vi "Instrument Identification.vi"() -> ()   [LabVIEW 2023]
doc: "Provides an example implementation of the Hardware Abstraction Framework to allow any attached instrument to be queried for its identity. The instrument must implement the SCPI standard.\n\nThe example application is clearly overly complex for the simple purpose of obtaining identity. However, it has been written to show how complex applications can be derived using the provided Event-Process-Result Handling mechanism. In fact, the base application can be reused by replacing the \"App ActionX Process\" VIs and \"Result Handling VIs\" as needed.\n\nNote that this example is just one way of interacting with the Framework. Ultimately, you just need to set up a Test Processor with what is needed and tell it to \"Process Directors\"."
uses:
  ReadCommand/ReadCommand.lvclass
  All Internal Message Ids.ctl
  ResourceEnumerator/ResourceEnumerator.lvclass
  CommandDirector/CommandDirector.lvclass
  TestProcessor/TestProcessor.lvclass
  <extravilib>/ChannelInstances/Tag-bool/Read With Abort.vi
  <extravilib>/ChannelInstances/Tag-bool/Write With Abort.vi
  <extravilib>/ChannelInstances/Tag-bool/Instantiate.vi
  <extravilib>/ChannelInstances/Tag-bool/EndpointRead.vi
  <extravilib>/ChannelInstances/Tag-bool/Endpoint.vi
  HAF.lvlib
  <extravilib>/ChannelInstances/Tag-bool.lvlib
panel:
  out "error out":errorcluster
  out "IDs":string[](array[string])
  out "Running":bool
  in  "Action10":bool
  in  "Action9":bool
  in  "Action8":bool
  in  "Action7":bool
  in  "Action6":bool
  in  "Action5":bool
  in  "Action4":bool
  in  "Action3":bool
  in  "Action2":bool
  in  "Instruments 2":string(combo)
  in  "Resume":bool
  in  "Pause":bool
  in  "Stop":bool
  in  "Get Id":bool caption="Action1"
  out "Instrument Id":string
  in  "Refresh":bool
  in  "Instruments":string(combo)
  # "Defined Behaviour Buttons"
  # "Instrument Identification"
  # "Re-usable Controls\n\nThese are hidden at runtime.  Unhide if used."
  # "Provides an example implementation of the Hardware Abstraction Framework to allow any attached instrument to be queried for its identity.  The instrument must implement the SCPI standard and must be defined in line with those in Implementation>Instrument.\n\nChoose an Instrument from the drop down list and click on Get Id.  The list can be refreshed by clicking Refresh.  The VI is terminated by clicking on Stop.\n\nThe example application is clearly overly complex for the simple purpose of obtaining identity.  However, it has been written to show how complex applications can be derived using the provided Event-Process-Result Handling mechanism.  In fact, the base application can be reused by replacing the \"App ActionX Process\" VIs and \"Result Handling VIs\" as needed.\n\nNote that this example is just one way of interacting with the Framework.  Ultimately, you just need to set up a Test Processor with what is needed and tell it to \"Process Directors\"."
  # "Defined Behaviour Buttons\n\nDrag the control from here to where needed.  You can relabel them but their behaviour is fixed in the application.\nYou may change this behaviour as well of course.\nStop and Refresh have been used."
  # "Instruments"
  # "Action Buttons"
  # "Instruments\n\nThese hold a list of Instruments attached to the PC and are populated by the \"Refresh\" Process case.  The Refresh button re-populates them."
  # "Action  Buttons\n\nDrag the control from here to where you need them on your panel.  Re-label and add button text as desired.\n\nPut processing code in the Process Case under their caption value.\n\nAction1 has been used and named \"Get Id\""
  # "Other"
  # "Other\n\nOther potentially useful controls or indicators. \nIDs is the collection of UUIDs generated for Commands during execution.\nThe LED Running is used in this example."
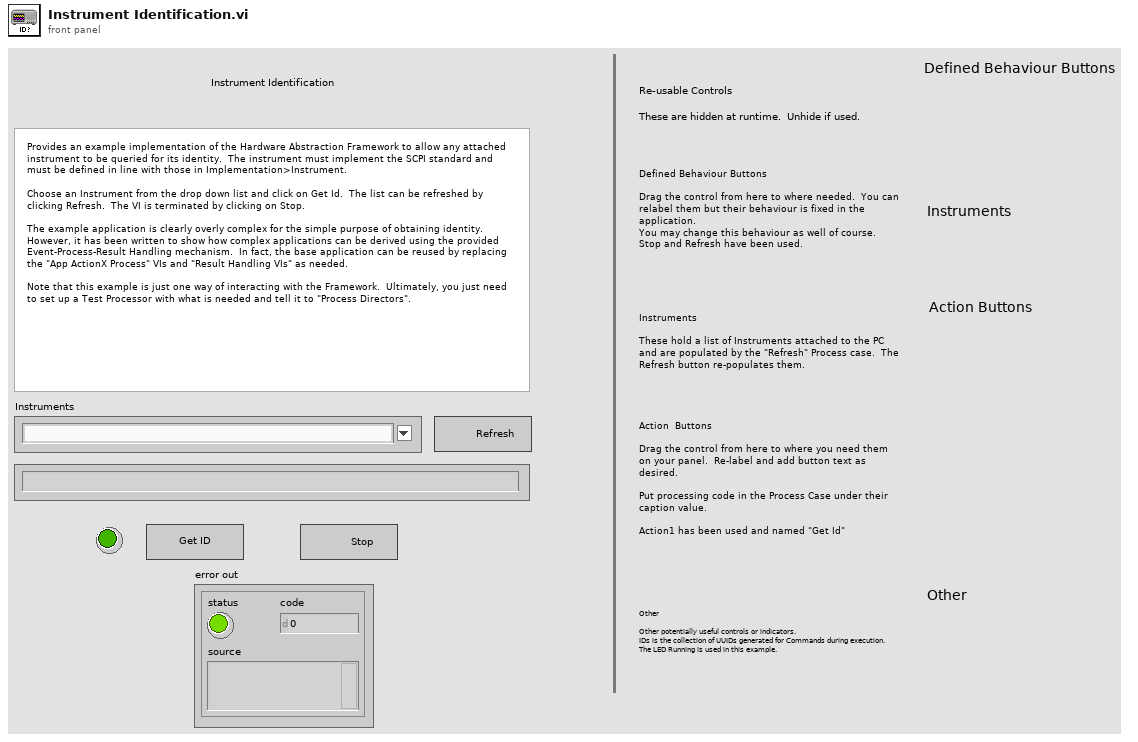
[diagram p1: front panel]
types:
  T1 = typedef "HAF.lvlib/All Message Queues.ctl" = cluster{"Internal":refnum<queue>, "Notifications":refnum<queue>}
  T2 = typedef "HAF.lvlib/All Events.ctl" = cluster{"Stop":T3, "Pause":T4, "Resume":T5, "Done":T6, "Injection":T7}
  T3 = typedef "HAF.lvlib/Stop Event.ctl" = refnum<user-event>
  T4 = typedef "HAF.lvlib/Pause Event.ctl" = refnum<user-event>
  T5 = typedef "HAF.lvlib/Resume Event.ctl" = refnum<user-event>
  T6 = typedef "HAF.lvlib/Done Event.ctl" = refnum<user-event>
  T7 = typedef "HAF.lvlib/Injection Event.ctl" = refnum<user-event>
  T8 = typedef "HAF.lvlib/All Internal Message Ids.ctl" = cluster{"Initialise":string, "Process":string, "Continue":string, "Done":string, "Pause":string, "Resume":string, "Stop":string, "Exit":string, "Inject":string}
  T9 = typedef "Tag-bool.lvlib/))Channel.ctl" = refnum<queue>
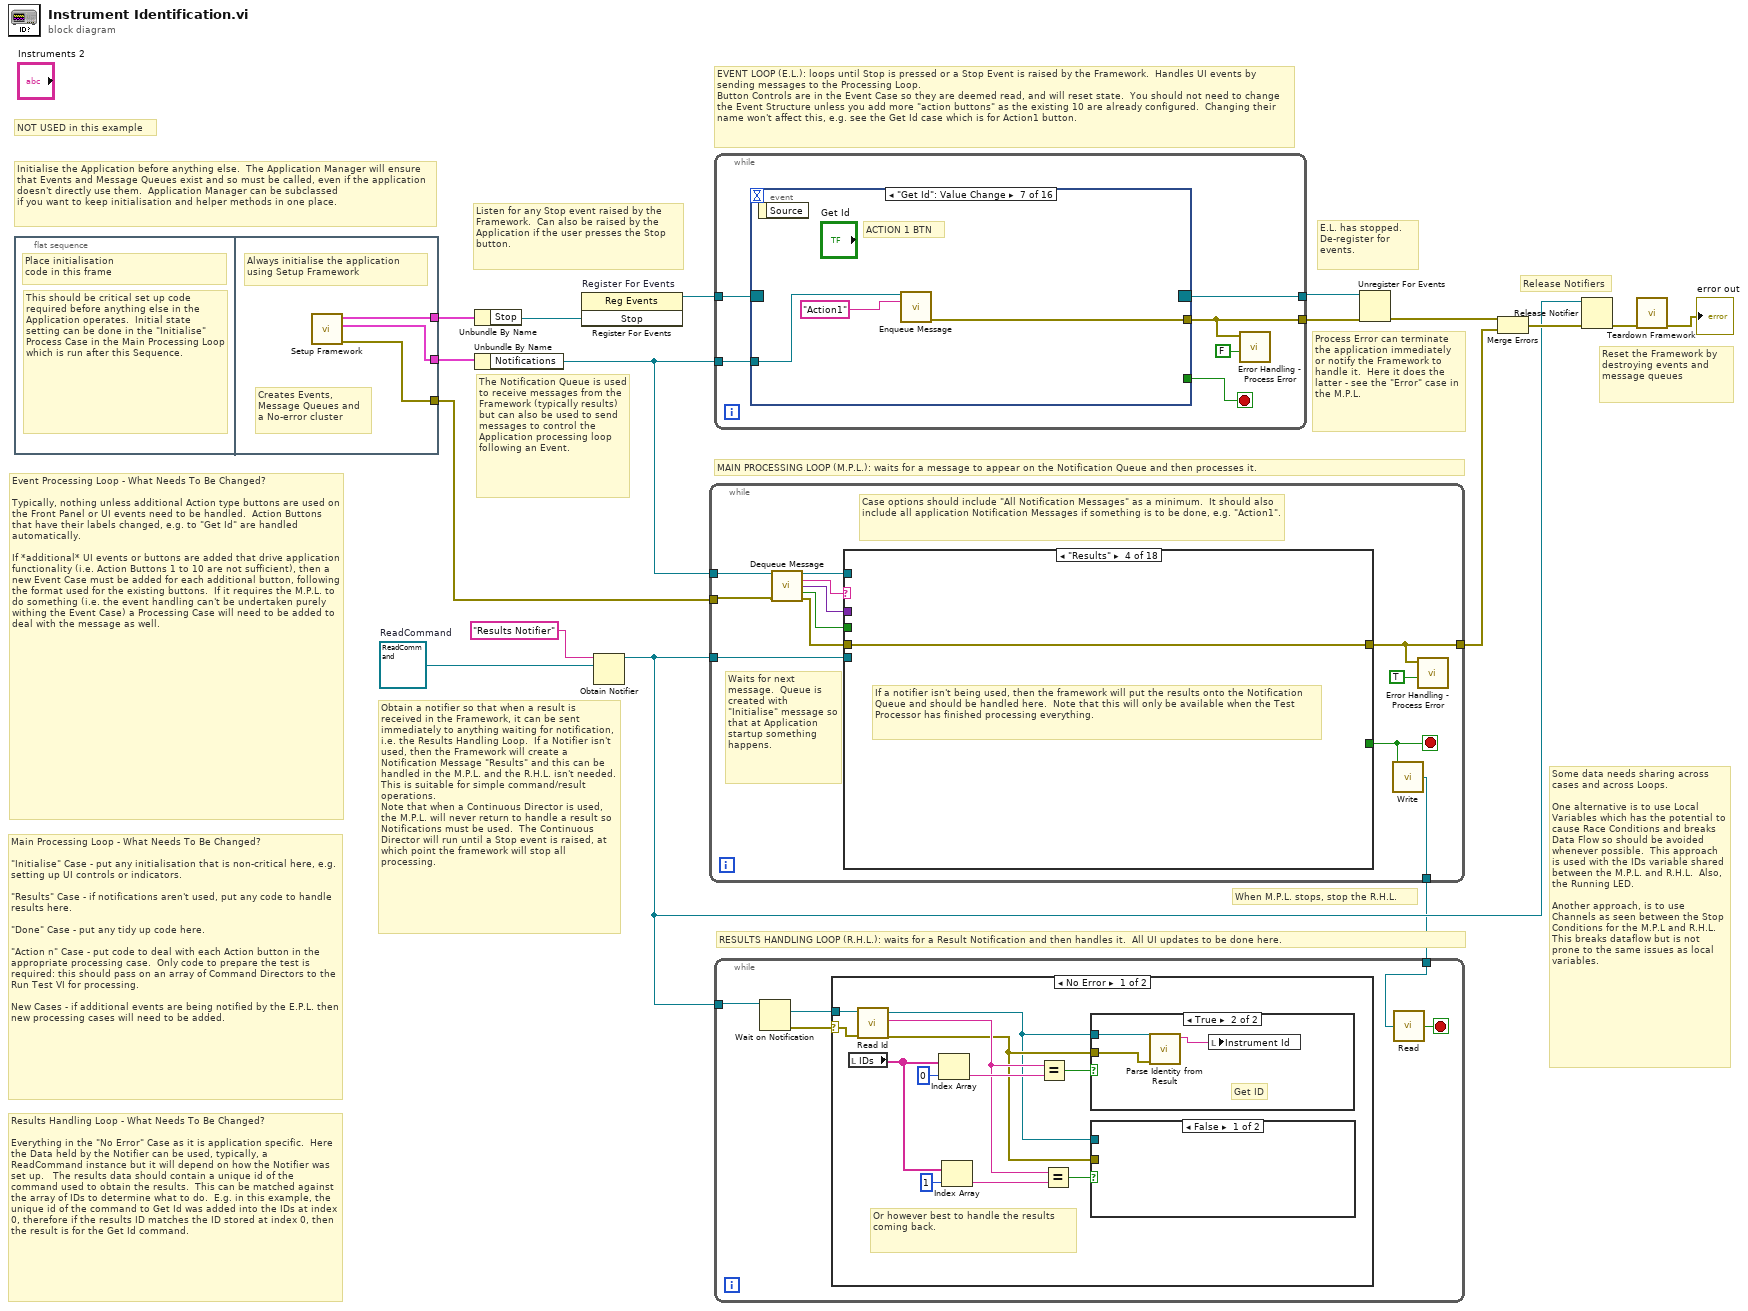
[diagram p0: block diagram]
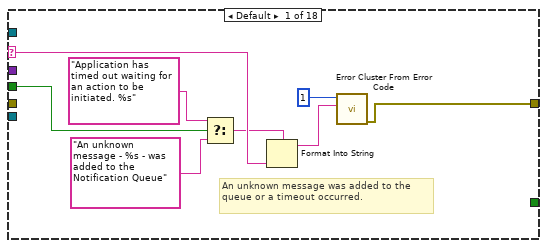
[diagram p5: hidden frame]
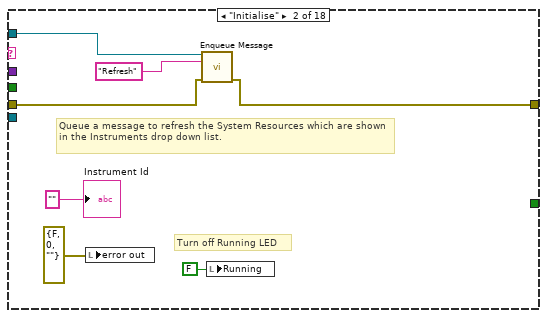
[diagram p6: hidden frame]
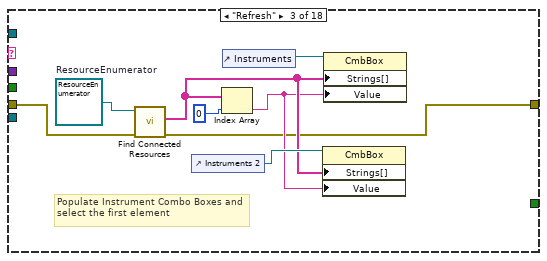
[diagram p7: hidden frame]
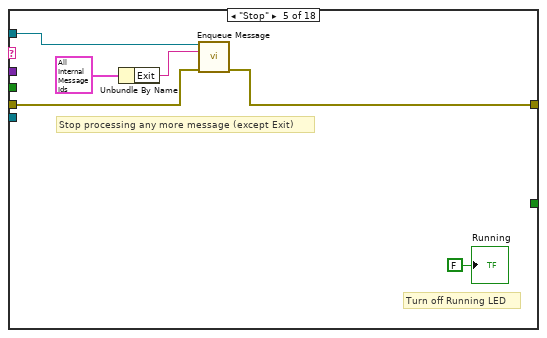
[diagram p8: hidden frame]
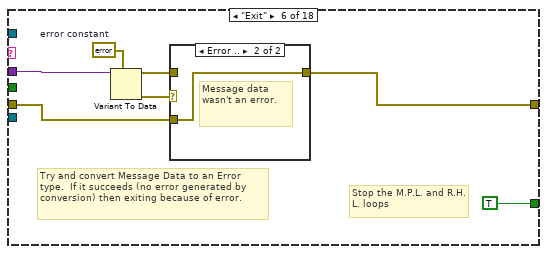
[diagram p9: hidden frame]
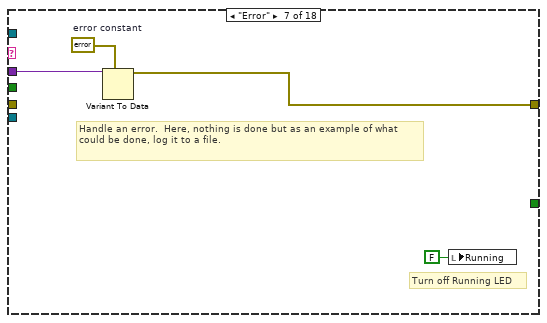
[diagram p11: hidden frame]
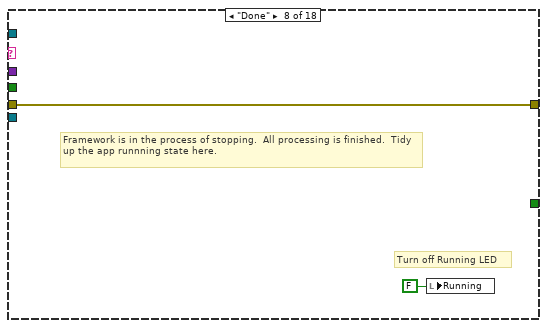
[diagram p12: hidden frame]
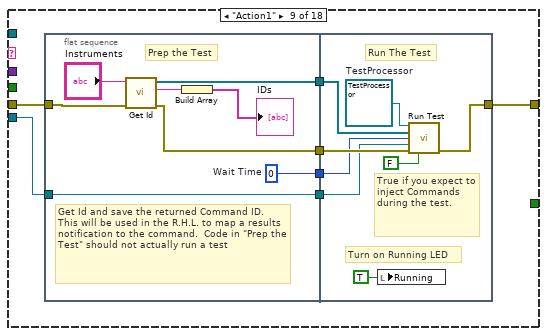
[diagram p13: hidden frame]
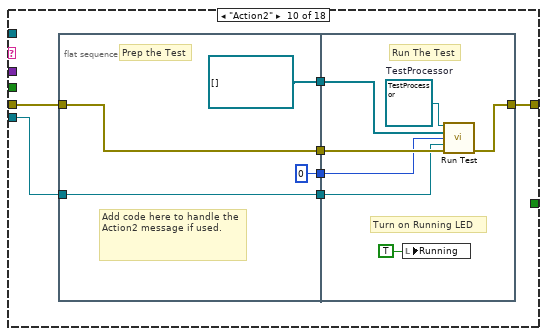
[diagram p14: hidden frame]
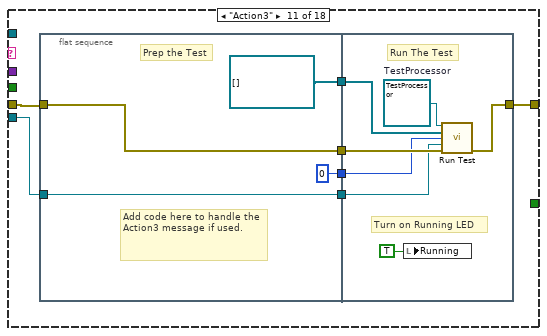
[diagram p15: hidden frame]
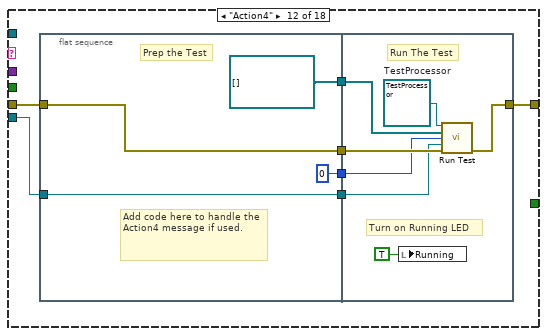
[diagram p16: hidden frame]
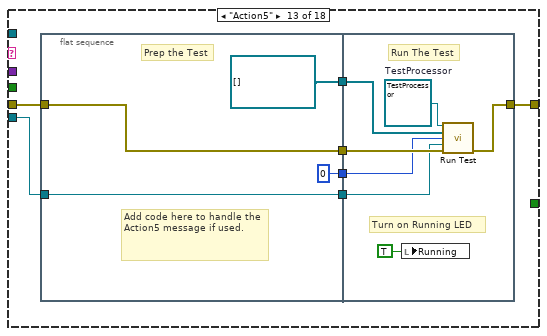
[diagram p17: hidden frame]
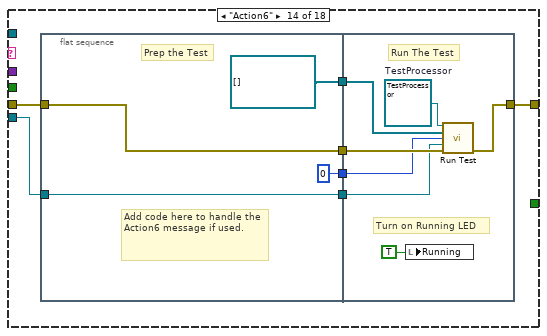
[diagram p18: hidden frame]
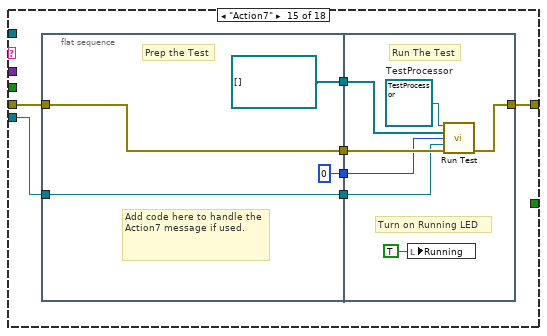
[diagram p19: hidden frame]
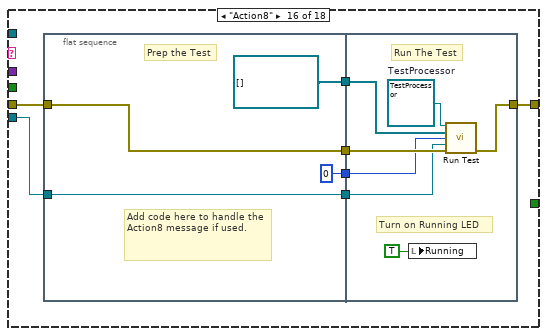
[diagram p20: hidden frame]
diagram:
  w8 = refnum<class "ReadCommand.lvclass"> refnum  # ReadCommand
  # "When M.P.L. stops, stop the R.H.L."
  # "Results Handling Loop - What Needs To Be Changed?\n\nEverything in the \"No Error\" Case as it is application specific.  Here the Data held by the Notifier can be used, typically, a ReadCommand instance but it will depend on how the Notifier was set up.   The results data should contain a unique id of the command used to obtain the results.  This can be matched against the array of IDs to determine what to do.  E.g. in this example, the unique id of the command to Get Id was added into the IDs at index 0, therefore if the results ID matches the ID stored at index 0, then the result is for the Get Id command."
  # "Reset the Framework by destroying events and message queues"
  # "Release Notifiers"
  # "Main Processing Loop - What Needs To Be Changed?\n\n\"Initialise\" Case - put any initialisation that is non-critical here, e.g. setting up UI controls or indicators.\n\n\"Results\" Case - if notifications aren't used, put any code to handle results here.\n\n\"Done\" Case - put any tidy up code here.\n\n\"Action n\" Case - put code to deal with each Action button in the appropriate processing case.  Only code to prepare the test is required: this should pass on an array of Command Directors to the Run Test VI for processing. \n\nNew Cases - if additional events are being notified by the E.P.L. then new processing cases will need to be added."
  # "Event Processing Loop - What Needs To Be Changed?\n\nTypically, nothing unless additional Action type buttons are used on the Front Panel or UI events need to be handled.  Action Buttons that have their labels changed, e.g. to \"Get Id\" are handled automatically.\n\nIf *additional* UI events or buttons are added that drive application functionality (i.e. Action Buttons 1 to 10 are not sufficient), then a new Event Case must be added for each additional button, following the format used for the existing buttons.  If it requires the M.P.L. to do something (i.e. the event handling can't be undertaken purely withing the Event Case) a Processing Case will need to be added to deal with the message as well."
  # "Some data needs sharing across cases and across Loops.\n\nOne alternative is to use Local Variables which has the potential to cause Race Conditions and breaks Data Flow so should be avoided whenever possible.  This approach is used with the IDs variable shared between the M.P.L. and R.H.L.  Also, the Running LED.\n\nAnother approach, is to use Channels as seen between the Stop Conditions for the M.P.L and R.H.L.  This breaks dataflow but is not prone to the same issues as local variables."
  # "Obtain a notifier so that when a result is received in the Framework, it can be sent immediately to anything waiting for notification, i.e. the Results Handling Loop.  If a Notifier isn't used, then the Framework will create a Notification Message \"Results\" and this can be handled in the M.P.L. and the R.H.L. isn't needed.  This is suitable for simple command/result operations.\nNote that when a Continuous Director is used, the M.P.L. will never return to handle a result so Notifications must be used.  The Continuous Director will run until a Stop event is raised, at which point the framework will stop all processing."
  # "Process Error can terminate the application immediately or notify the Framework to handle it.  Here it does the latter - see the \"Error\" case in the M.P.L."
  # "E.L. has stopped.  De-register for events."
  # "RESULTS HANDLING LOOP (R.H.L.): waits for a Result Notification and then handles it.  All UI updates to be done here."
  # "MAIN PROCESSING LOOP (M.P.L.): waits for a message to appear on the Notification Queue and then processes it."
  # "EVENT LOOP (E.L.): loops until Stop is pressed or a Stop Event is raised by the Framework.  Handles UI events by sending messages to the Processing Loop.\nButton Controls are in the Event Case so they are deemed read, and will reset state.  You should not need to change the Event Structure unless you add more \"action buttons\" as the existing 10 are already configured.  Changing their name won't affect this, e.g. see the Get Id case which is for Action1 button."
  # "NOT USED in this example"
  # "Listen for any Stop event raised by the Framework.  Can also be raised by the Application if the user presses the Stop button."
  # "The Notification Queue is used to receive messages from the Framework (typically results) but can also be used to send messages to control the Application processing loop following an Event."
  # "Initialise the Application before anything else.  The Application Manager will ensure that Events and Message Queues exist and so must be called, even if the application doesn't directly use them.  Application Manager can be subclassed\nif you want to keep initialisation and helper methods in one place."
  n1 = flat-sequence {
    tunnel: [w20] -> w16
    tunnel: [w19] -> w17
    tunnel: [w18] -> w10
    frame #0 {
      # "This should be critical set up code required before anything else in the Application operates.  Initial state setting can be done in the \"Initialise\" Process Case in the Main Processing Loop which is run after this Sequence."
      # "Place initialisation\ncode in this frame"
    }
    frame #1 {
      # "Creates Events,  \nMessage Queues and\na No-error cluster"
      # "Always initialise the application using Setup Framework"
      n2 = call "Setup Framework.vi"() -> ("error out"=w18:errorcluster, "Message Queues"=w19:T1, "Events"=w20:T2)  [unwired: 9 in]
    }
  }
  n3 = Unbundle By Name(w16) -> ("Stop"=w14:T3)
  n4 = Unbundle By Name(w17) -> ("Notifications"=w11:refnum<queue>)
  n5 = register-events "Register For Events"(w14) -> (reference out=w15:refnum<event-registration>)  [unwired: 2 in, 1 out]
  n6 = Obtain Notifier(name (unnamed)="Results Notifier", notification data type=w8) -> (notifier out=w4:refnum<notifier>)  [unwired: 2 in, 2 out]
  n7 = while {
    tunnel: w11 -> [w32]
    tunnel: w10 -> [w31]
    tunnel: w4 -> [w25]
    tunnel: [w24] -> w6
    tunnel: [w21] -> w1
    stop <- w22 stop-if-true
    # "Case options should include \"All Notification Messages\" as a minimum.  It should also include all application Notification Messages if something is to be done, e.g. \"Action1\"."
    # "Waits for next message.  Queue is created with \"Initialise\" message so that at Application startup something happens."
    n8 = call "Dequeue Message.vi"("Message Queue In"=w32, "error in (no error)"=w31) -> ("Message Queue Out"=w30:refnum<queue>, "Message Id"=w29:string, "Message Data"=w28:variant, "Timed Out"=w26:bool, "error out"=w27:errorcluster)  [unwired: 9 in]
    n9 = case shown="\"Results\"" w29 {
      selector: w29 -> [w37 _ _ _ _ _ _ _ _ _ _ _ _ _ _ _ _ _]
      tunnel: w30 -> [_ w47 _ _ w62 _ _ _ _ _ _ _ _ _ _ _ _ _]
      tunnel: w28 -> [_ _ _ _ _ w69 w75 _ _ _ _ _ _ _ _ _ _ _]
      tunnel: w27 -> [_ w45 w54 w56 w59 w65 _ w77 w83 w103 w120 w137 w156 w174 w192 w210 w229 w246]
      tunnel: w26 -> [w39 _ _ _ _ _ _ _ _ _ _ _ _ _ _ _ _ _]
      tunnel: w25 -> [_ _ _ _ _ _ _ _ w84 w102 w119 w138 w155 w173 w191 w209 w228 w245]
      tunnel: [w33 w44 w48 w56 w58 w66 w74 w77 w82 w101 w121 w139 w157 w175 w193 w211 w227 w247] -> w24
      tunnel: [_ _ _ _ _ TRUE ("Running") _ _ _ _ _ _ _ _ _ _ _ _] -> w22
      frame Default {
        # "An unknown message was added to the queue or a timeout occurred."
        n10 = Select(t="Application has timed out waiting for an action to be initiated. %s", s=w39, f="An unknown message - %s - was added to the Notification Queue") -> (s? t:f=w36:string)
        n11 = Format Into String(format string=w36, w37) -> (resulting string=w34:string)  [unwired: 2 in, 1 out]
        n12 = call <vilib>:"Error Cluster From Error Code.vi"("error message (\"\")"=w34, "error code (0)"=1) -> ("error out"=w33:errorcluster)  [unwired: 7 in]
      }
      frame "Initialise" {
        # "Turn off Running LED"
        # "Queue a message to refresh the System Resources which are shown in the Instruments drop down list."
        n13 = local write "error out"(errorcluster {"status"=FALSE, "code"=0, "source"=""} ("error constant")) -> ()
        n14 = call "Enqueue Message.vi"("Message Queue In"=w47, "Message Id"="Refresh", "error in (no error)"=w45) -> ("error out"=w44:errorcluster)  [unwired: 11 in, 1 out]
        n15 = local write "Running"(FALSE ("Running")) -> ()
        "Instrument Id" <- "" ("Instrument Id")
      }
      frame "Refresh" {
        w55 = refnum<class "ResourceEnumerator.lvclass"> refnum  # ResourceEnumerator
        # "Populate Instrument Combo Boxes and select the first element"
        n16 = call-dynamic "Find Connected Resources.vi"("error in (no error)"=w54, "AbstractResourceEnumerator in"=w55) -> ("error out"=w48:errorcluster, "Found Resources"=w50:string[])  [unwired: 7 in, 1 out]
        n17 = control-ref of="Instruments 2"() -> (w51:refnum<vi>)
        n18 = Index Array(array=w50, index=0) -> (element=w49:string)
        n19 = control-ref of="Instruments"() -> (w53:refnum<vi>)
        n20 = property class="CmbBox"(reference=w51, "Strings[]"=w50, "Value"=w49) -> ()  [unwired: 1 in, 2 out]
        n21 = property class="CmbBox"(reference=w53, "Strings[]"=w50, "Value"=w49) -> ()  [unwired: 1 in, 2 out]
      }
      frame "Results" {
        # "If a notifier isn't being used, then the framework will put the results onto the Notification Queue and should be handled here.  Note that this will only be available when the Test Processor has finished processing everything."
      }
      frame "Stop" {
        # "Stop processing any more message (except Exit)"
        # "Turn off Running LED"
        n22 = Unbundle By Name(T8 {"Initialise"="Initialise", "Process"="Process", "Continue"="Continue", "Done"="Done", "Pause"="Pause", "Resume"="Resume", "Stop"="Stop", "Exit"="Exit", "Inject"=""} ("Message Ids")) -> ("Exit"=w60:string)
        n23 = call "Enqueue Message.vi"("Message Queue In"=w62, "Message Id"=w60, "error in (no error)"=w59) -> ("error out"=w58:errorcluster)  [unwired: 11 in, 1 out]
        "Running" <- FALSE ("Running")
      }
      frame "Exit" {
        w64 = errorcluster {"status"=FALSE, "code"=0, "source"=""}  # error constant
        # "Try and convert Message Data to an Error type.  If it succeeds (no error generated by conversion) then exiting because of error."
        # "Stop the M.P.L. and R.H.L. loops"
        n24 = Variant To Data(type=w64, Variant=w69) -> (data=w67:errorcluster, error out=w68:errorcluster)  [unwired: 1 in]
        n25 = case shown="Error .." w68 {
          tunnel: w67 -> [w70 _]
          tunnel: [w70 w71] -> w66
          tunnel: w65 -> [_ w71]
          frame No Error {
            # "If exiting because of error, pass it on for display"
          }
          frame Error {
            # "Message data wasn't an error."
          }
        }
      }
      frame "Error" {
        w73 = errorcluster {"status"=FALSE, "code"=0, "source"=""}  # error constant
        # "Turn off Running LED"
        # "Handle an error.  Here, nothing is done but as an example of what could be done, log it to a file."
        n26 = Variant To Data(type=w73, Variant=w75) -> (data=w74:errorcluster)  [unwired: 1 in, 1 out]
        n27 = local write "Running"(FALSE ("Running")) -> ()
      }
      frame "Done" {
        # "Turn off Running LED"
        # "Framework is in the process of stopping.  All processing is finished.  Tidy up the app runnning state here."
        n28 = local write "Running"(FALSE ("Running")) -> ()
      }
      frame "Action1" {
        n29 = flat-sequence {
          tunnel: w84 -> [w86]
          tunnel: w83 -> [w91]
          tunnel: [w90] -> w81
          tunnel: [w87] -> w80
          tunnel: [w86] -> w79
          tunnel: [w85] -> w78
          tunnel: [w99] -> w82
          tunnel: w81 -> [w97]
          tunnel: w80 -> [w98]
          tunnel: w79 -> [w96]
          tunnel: w78 -> [w95]
          frame #0 {
            w85 = u32 0  # Wait Time
            # "Get Id and save the returned Command ID.  This will be used in the R.H.L. to map a results notification to the command.  Code in \"Prep the Test\" should not actually run a test"
            # "Prep the Test"
            n30 = call "Get Id.vi"("error in (no error)"=w91, "Instrument Name"="Instruments") -> ("error out"=w90:errorcluster, "ID of IDN Command"=w88:string, "CommandDirectors"=w87:refnum<class "CommandDirector.lvclass">[])  [unwired: 6 in]
            n31 = Build Array(w88) -> (→"IDs":string[])
          }
          frame #1 {
            w100 = refnum<class "TestProcessor.lvclass"> refnum  # TestProcessor
            # "True if you expect to inject Commands during the test."
            # "Turn on Running LED"
            # "Run The Test"
            n32 = local write "Running"(TRUE ("Running")) -> ()
            n33 = call-dynamic "Run Test.vi"("TestProcessor in"=w100, "Command Directors"=w98, "Wait Time"=w95, "Results Notifier"=w96, "error in (no error)"=w97, "Handle Injections"=FALSE) -> ("error out"=w99:errorcluster)  [unwired: 8 in, 1 out]
          }
        }
      }
      frame "Action2" {
        n34 = flat-sequence {
          tunnel: w102 -> [w111]
          tunnel: w103 -> [w110]
          tunnel: [w110] -> w107
          tunnel: [refnum<class "CommandDirector.lvclass">[] [] ("CommandDirectors")] -> w106
          tunnel: [w111] -> w105
          tunnel: [u32 0 ("Wait Time")] -> w104
          tunnel: [w117] -> w101
          tunnel: w107 -> [w115]
          tunnel: w106 -> [w116]
          tunnel: w105 -> [w114]
          tunnel: w104 -> [w113]
          frame #0 {
            # "Add code here to handle the Action2 message if used."
            # "Prep the Test"
          }
          frame #1 {
            w118 = refnum<class "TestProcessor.lvclass"> refnum  # TestProcessor
            # "Turn on Running LED"
            # "Run The Test"
            n35 = local write "Running"(TRUE ("Running")) -> ()
            n36 = call-dynamic "Run Test.vi"("TestProcessor in"=w118, "Command Directors"=w116, "Wait Time"=w113, "Results Notifier"=w114, "error in (no error)"=w115) -> ("error out"=w117:errorcluster)  [unwired: 9 in, 1 out]
          }
        }
      }
      frame "Action3" {
        n37 = flat-sequence {
          tunnel: w119 -> [w129]
          tunnel: w120 -> [w128]
          tunnel: [w128] -> w125
          tunnel: [refnum<class "CommandDirector.lvclass">[] [] ("CommandDirectors")] -> w124
          tunnel: [w129] -> w123
          tunnel: [u32 0 ("Wait Time")] -> w122
          tunnel: [w135] -> w121
          tunnel: w125 -> [w133]
          tunnel: w124 -> [w134]
          tunnel: w123 -> [w132]
          tunnel: w122 -> [w131]
          frame #0 {
            # "Add code here to handle the Action3 message if used."
            # "Prep the Test"
          }
          frame #1 {
            w136 = refnum<class "TestProcessor.lvclass"> refnum  # TestProcessor
            # "Turn on Running LED"
            # "Run The Test"
            n38 = local write "Running"(TRUE ("Running")) -> ()
            n39 = call-dynamic "Run Test.vi"("TestProcessor in"=w136, "Command Directors"=w134, "Wait Time"=w131, "Results Notifier"=w132, "error in (no error)"=w133) -> ("error out"=w135:errorcluster)  [unwired: 9 in, 1 out]
          }
        }
      }
      frame "Action4" {
        n40 = flat-sequence {
          tunnel: w138 -> [w147]
          tunnel: w137 -> [w146]
          tunnel: [w146] -> w143
          tunnel: [refnum<class "CommandDirector.lvclass">[] [] ("CommandDirectors")] -> w142
          tunnel: [w147] -> w141
          tunnel: [u32 0 ("Wait Time")] -> w140
          tunnel: [w153] -> w139
          tunnel: w143 -> [w151]
          tunnel: w142 -> [w152]
          tunnel: w141 -> [w150]
          tunnel: w140 -> [w149]
          frame #0 {
            # "Add code here to handle the Action4 message if used."
            # "Prep the Test"
          }
          frame #1 {
            w154 = refnum<class "TestProcessor.lvclass"> refnum  # TestProcessor
            # "Turn on Running LED"
            # "Run The Test"
            n41 = local write "Running"(TRUE ("Running")) -> ()
            n42 = call-dynamic "Run Test.vi"("TestProcessor in"=w154, "Command Directors"=w152, "Wait Time"=w149, "Results Notifier"=w150, "error in (no error)"=w151) -> ("error out"=w153:errorcluster)  [unwired: 9 in, 1 out]
          }
        }
      }
      frame "Action5" {
        n43 = flat-sequence {
          tunnel: w155 -> [w165]
          tunnel: w156 -> [w164]
          tunnel: [w164] -> w161
          tunnel: [refnum<class "CommandDirector.lvclass">[] [] ("CommandDirectors")] -> w160
          tunnel: [w165] -> w159
          tunnel: [u32 0 ("Wait Time")] -> w158
          tunnel: [w171] -> w157
          tunnel: w161 -> [w169]
          tunnel: w160 -> [w170]
          tunnel: w159 -> [w168]
          tunnel: w158 -> [w167]
          frame #0 {
            # "Add code here to handle the Action5 message if used."
            # "Prep the Test"
          }
          frame #1 {
            w172 = refnum<class "TestProcessor.lvclass"> refnum  # TestProcessor
            # "Turn on Running LED"
            # "Run The Test"
            n44 = local write "Running"(TRUE ("Running")) -> ()
            n45 = call-dynamic "Run Test.vi"("TestProcessor in"=w172, "Command Directors"=w170, "Wait Time"=w167, "Results Notifier"=w168, "error in (no error)"=w169) -> ("error out"=w171:errorcluster)  [unwired: 9 in, 1 out]
          }
        }
      }
      frame "Action6" {
        n46 = flat-sequence {
          tunnel: w173 -> [w183]
          tunnel: w174 -> [w182]
          tunnel: [w182] -> w179
          tunnel: [refnum<class "CommandDirector.lvclass">[] [] ("CommandDirectors")] -> w178
          tunnel: [w183] -> w177
          tunnel: [u32 0 ("Wait Time")] -> w176
          tunnel: [w189] -> w175
          tunnel: w179 -> [w187]
          tunnel: w178 -> [w188]
          tunnel: w177 -> [w186]
          tunnel: w176 -> [w185]
          frame #0 {
            # "Add code here to handle the Action6 message if used."
            # "Prep the Test"
          }
          frame #1 {
            w190 = refnum<class "TestProcessor.lvclass"> refnum  # TestProcessor
            # "Turn on Running LED"
            # "Run The Test"
            n47 = local write "Running"(TRUE ("Running")) -> ()
            n48 = call-dynamic "Run Test.vi"("TestProcessor in"=w190, "Command Directors"=w188, "Wait Time"=w185, "Results Notifier"=w186, "error in (no error)"=w187) -> ("error out"=w189:errorcluster)  [unwired: 9 in, 1 out]
          }
        }
      }
      frame "Action7" {
        n49 = flat-sequence {
          tunnel: w191 -> [w201]
          tunnel: w192 -> [w200]
          tunnel: [w200] -> w197
          tunnel: [refnum<class "CommandDirector.lvclass">[] [] ("CommandDirectors")] -> w196
          tunnel: [w201] -> w195
          tunnel: [u32 0 ("Wait Time")] -> w194
          tunnel: [w207] -> w193
          tunnel: w197 -> [w205]
          tunnel: w196 -> [w206]
          tunnel: w195 -> [w204]
          tunnel: w194 -> [w203]
          frame #0 {
            # "Add code here to handle the Action7 message if used."
            # "Prep the Test"
          }
          frame #1 {
            w208 = refnum<class "TestProcessor.lvclass"> refnum  # TestProcessor
            # "Turn on Running LED"
            # "Run The Test"
            n50 = local write "Running"(TRUE ("Running")) -> ()
            n51 = call-dynamic "Run Test.vi"("TestProcessor in"=w208, "Command Directors"=w206, "Wait Time"=w203, "Results Notifier"=w204, "error in (no error)"=w205) -> ("error out"=w207:errorcluster)  [unwired: 9 in, 1 out]
          }
        }
      }
      frame "Action8" {
        n52 = flat-sequence {
          tunnel: w209 -> [w219]
          tunnel: w210 -> [w218]
          tunnel: [w218] -> w215
          tunnel: [refnum<class "CommandDirector.lvclass">[] [] ("CommandDirectors")] -> w214
          tunnel: [w219] -> w213
          tunnel: [u32 0 ("Wait Time")] -> w212
          tunnel: [w225] -> w211
          tunnel: w215 -> [w223]
          tunnel: w214 -> [w224]
          tunnel: w213 -> [w222]
          tunnel: w212 -> [w221]
          frame #0 {
            # "Add code here to handle the Action8 message if used."
            # "Prep the Test"
          }
          frame #1 {
            w226 = refnum<class "TestProcessor.lvclass"> refnum  # TestProcessor
            # "Turn on Running LED"
            # "Run The Test"
            n53 = local write "Running"(TRUE ("Running")) -> ()
            n54 = call-dynamic "Run Test.vi"("TestProcessor in"=w226, "Command Directors"=w224, "Wait Time"=w221, "Results Notifier"=w222, "error in (no error)"=w223) -> ("error out"=w225:errorcluster)  [unwired: 9 in, 1 out]
          }
        }
      }
      frame "Action9" {
        n55 = flat-sequence {
          tunnel: w228 -> [w237]
          tunnel: w229 -> [w236]
          tunnel: [w236] -> w233
          tunnel: [refnum<class "CommandDirector.lvclass">[] [] ("CommandDirectors")] -> w232
          tunnel: [w237] -> w231
          tunnel: [u32 0 ("Wait Time")] -> w230
          tunnel: w233 -> [w242]
          tunnel: w232 -> [w243]
          tunnel: w231 -> [w241]
          tunnel: w230 -> [w240]
          tunnel: [w239] -> w227
          frame #0 {
            # "Add code here to handle the Action9 message if used."
            # "Prep the Test"
          }
          frame #1 {
            w244 = refnum<class "TestProcessor.lvclass"> refnum  # TestProcessor
            # "Turn on Running LED"
            # "Run The Test"
            n56 = local write "Running"(TRUE ("Running")) -> ()
            n57 = call-dynamic "Run Test.vi"("TestProcessor in"=w244, "Command Directors"=w243, "Wait Time"=w240, "Results Notifier"=w241, "error in (no error)"=w242) -> ("error out"=w239:errorcluster)  [unwired: 9 in, 1 out]
          }
        }
      }
      frame "Action10" {
        n58 = flat-sequence {
          tunnel: w245 -> [w255]
          tunnel: w246 -> [w254]
          tunnel: [w254] -> w251
          tunnel: [refnum<class "CommandDirector.lvclass">[] [] ("CommandDirectors")] -> w250
          tunnel: [w255] -> w249
          tunnel: [u32 0 ("Wait Time")] -> w248
          tunnel: [w261] -> w247
          tunnel: w251 -> [w259]
          tunnel: w250 -> [w260]
          tunnel: w249 -> [w258]
          tunnel: w248 -> [w257]
          frame #0 {
            # "Add code here to handle the Action10 message if used."
            # "Prep the Test"
          }
          frame #1 {
            w262 = refnum<class "TestProcessor.lvclass"> refnum  # TestProcessor
            # "Turn on Running LED"
            # "Run The Test"
            n59 = local write "Running"(TRUE ("Running")) -> ()
            n60 = call-dynamic "Run Test.vi"("TestProcessor in"=w262, "Command Directors"=w260, "Wait Time"=w257, "Results Notifier"=w258, "error in (no error)"=w259) -> ("error out"=w261:errorcluster)  [unwired: 9 in, 1 out]
          }
        }
      }
    }
    n61 = call <extravilib>:"Write.vi"("element"=w22) -> ("channel"=w21:T9)  [unwired: 1 out]
    n62 = call "Error Handling - Process Error.vi"("Exit on Error"=TRUE, "error to process"=w24) -> ()  [unwired: 9 in, 1 out]
  }
  n63 = while {
    tunnel: w11 -> [w267]
    tunnel: w15 -> [w268]
    tunnel: [w265] -> w13
    tunnel: [w264] -> w12
    stop <- w266 stop-if-true
    n64 = event shown="[6] \"Get Id\": Value Change" {
      selector: w268 -> [_ _ _ _ _ _ _ _ _ _ _ _ _ _ _ _]
      dyn-events: [_ _ _ _ _ _ _ _ _ _ _ _ _ _ _ _] -> w265
      timeout: _ -> [_ _ _ _ _ _ _ _ _ _ _ _ _ _ _ _]
      tunnel: w267 -> [_ w271 _ _ w281 _ w289 w291 w294 w297 w300 w303 w306 w309 w312 w315]
      tunnel: [_ w269 w272 w275 w279 w284 w287 w290 w293 w296 w299 w302 w305 w308 w311 w314] -> w264
      tunnel: [_ _ _ _ TRUE _ _ _ _ _ _ _ _ _ _ _] -> w266
      event Timeout {
        n65 = event-data() -> ()  [unwired: 1 in, 3 out]
      }
      event "Refresh": Value Change {
        # "Notify M.P.L. to rebuild attached instruments"
        n66 = event-data() -> ()  [unwired: 1 in, 1 out]
        n67 = call "Enqueue Message.vi"("Message Queue In"=w271, "Message Id"="Refresh") -> ("error out"=w269:errorcluster)  [unwired: 12 in, 1 out]
      }
      event "Pause": Value Change {
        # "Tell the Framework to Pause processing."
        n68 = event-data() -> ()  [unwired: 1 in, 1 out]
        n69 = call "Raise Pause Event.vi"("Raiser Name"="Instrument Identification", "Send Pause"=TRUE) -> ("error out"=w272:errorcluster)  [unwired: 8 in]
      }
      event "Resume": Value Change {
        # "Tell the Framework to Resume processing."
        n70 = event-data() -> ()  [unwired: 1 in, 1 out]
        n71 = call "Raise Resume Event.vi"("Send Resume"=TRUE, "Raiser Name"="Instrument Identification") -> ("error out"=w275:errorcluster)  [unwired: 9 in]
      }
      event User Event {
        # "Tell M.P.L. to stop processsing, high priority.  Exit Event Loop."
        n72 = event-data() -> ()  [unwired: 1 in, 1 out]
        n73 = Unbundle By Name(T8 {"Initialise"="Initialise", "Process"="Process", "Continue"="Continue", "Done"="Done", "Pause"="Pause", "Resume"="Resume", "Stop"="Stop", "Exit"="Exit", "Inject"=""} ("Message Ids")) -> ("Stop"=w282:string)
        n74 = call "Enqueue Message.vi"("Message Queue In"=w281, "Message Id"=w282, "Priority"=TRUE) -> ("error out"=w279:errorcluster)  [unwired: 11 in, 1 out]
      }
      event "Stop": Value Change {
        # "When Stop pressed, raise Stop Event to halt further processing"
        n75 = event-data() -> ()  [unwired: 1 in, 1 out]
        n76 = call "Raise Stop Event.vi"("Send Stop"=TRUE, "Raiser Name"="Instrument Identification") -> ("error out"=w284:errorcluster)  [unwired: 9 in]
      }
      event "Get Id": Value Change {
        # "ACTION 1 BTN"
        n77 = event-data() -> ()  [unwired: 1 in, 1 out]
        n78 = call "Enqueue Message.vi"("Message Queue In"=w289, "Message Id"="Action1") -> ("error out"=w287:errorcluster)  [unwired: 12 in, 1 out]
      }
      event "Action2": Value Change {
        # "ACTION 2 BTN"
        n79 = event-data() -> ()  [unwired: 1 in, 1 out]
        n80 = call "Enqueue Message.vi"("Message Queue In"=w291, "Message Id"="Action2") -> ("error out"=w290:errorcluster)  [unwired: 12 in, 1 out]
      }
      event "Action3": Value Change {
        # "ACTION 3 BTN"
        n81 = event-data() -> ()  [unwired: 1 in, 1 out]
        n82 = call "Enqueue Message.vi"("Message Queue In"=w294, "Message Id"="Action3") -> ("error out"=w293:errorcluster)  [unwired: 12 in, 1 out]
      }
      event "Action4": Value Change {
        # "ACTION 4 BTN"
        n83 = event-data() -> ()  [unwired: 1 in, 1 out]
        n84 = call "Enqueue Message.vi"("Message Queue In"=w297, "Message Id"="Action4") -> ("error out"=w296:errorcluster)  [unwired: 12 in, 1 out]
      }
      event "Action5": Value Change {
        # "ACTION 5 BTN"
        n85 = event-data() -> ()  [unwired: 1 in, 1 out]
        n86 = call "Enqueue Message.vi"("Message Queue In"=w300, "Message Id"="Action5") -> ("error out"=w299:errorcluster)  [unwired: 12 in, 1 out]
      }
      event "Action6": Value Change {
        # "ACTION 6 BTN"
        n87 = event-data() -> ()  [unwired: 1 in, 1 out]
        n88 = call "Enqueue Message.vi"("Message Queue In"=w303, "Message Id"="Action6") -> ("error out"=w302:errorcluster)  [unwired: 12 in, 1 out]
      }
      event "Action7": Value Change {
        # "ACTION 7 BTN"
        n89 = event-data() -> ()  [unwired: 1 in, 1 out]
        n90 = call "Enqueue Message.vi"("Message Queue In"=w306, "Message Id"="Action7") -> ("error out"=w305:errorcluster)  [unwired: 12 in, 1 out]
      }
      event "Action8": Value Change {
        # "ACTION 8 BTN"
        n91 = event-data() -> ()  [unwired: 1 in, 1 out]
        n92 = call "Enqueue Message.vi"("Message Queue In"=w309, "Message Id"="Action8") -> ("error out"=w308:errorcluster)  [unwired: 12 in, 1 out]
      }
      event "Action9": Value Change {
        # "ACTION 9 BTN"
        n93 = event-data() -> ()  [unwired: 1 in, 1 out]
        n94 = call "Enqueue Message.vi"("Message Queue In"=w312, "Message Id"="Action9") -> ("error out"=w311:errorcluster)  [unwired: 12 in, 1 out]
      }
      event "Action10": Value Change {
        # "ACTION 10 BTN"
        n95 = event-data() -> ()  [unwired: 1 in, 1 out]
        n96 = call "Enqueue Message.vi"("Message Queue In"=w315, "Message Id"="Action1") -> ("error out"=w314:errorcluster)  [unwired: 12 in, 1 out]
      }
    }
    n97 = call "Error Handling - Process Error.vi"("Exit on Error"=FALSE, "error to process"=w264) -> ()  [unwired: 9 in, 1 out]
  }
  n98 = while {
    tunnel: w4 -> [w321]
    tunnel: w1 -> [w317]
    stop <- w318 stop-if-true
    n99 = Wait on Notification(notifier=w321) -> (notification=w320:refnum<class "ReadCommand.lvclass">, error out=w319:errorcluster)  [unwired: 3 in, 2 out]
    n100 = case shown="No Error" w319 {
      selector: w319 -> [w329 _]
      tunnel: w320 -> [w333 _]
      frame No Error {
        # "Or however best to handle the results coming back."
        n101 = local read "IDs"() -> (w324:string[])
        n102 = call-dynamic "Read Id.vi"("error in (no error)"=w329, "WriteCommand in"=w333) -> ("error out"=w323:errorcluster, "Id"=w325:string, "WriteCommand out"=w322:refnum<class "ReadCommand.lvclass">)  [unwired: 7 in]
        n103 = Index Array(array=w324, index=0) -> (element=w331:string)
        n104 = Index Array(array=w324, index=1) -> (element=w326:string)
        n105 = Equal?(x=w325, y=w331) -> (x = y?=w330:bool)
        n106 = Equal?(x=w325, y=w326) -> (x = y?=w327:bool)
        n107 = case shown="True" w330 {
          tunnel: w322 -> [_ w336]
          tunnel: w323 -> [_ w335]
          frame False {
          }
          frame True {
            # "Get ID"
            n108 = call "Parse Identity from Result.vi"("error in (no error)"=w335, "ReadCommand In"=w336) -> ("Identity"=w334:string)  [unwired: 8 in, 1 out]
            n109 = local write "Instrument Id"(w334) -> ()
          }
        }
        n110 = case shown="False" w327 {
          tunnel: w323 -> [_ _]
          tunnel: w322 -> [_ _]
          frame False {
          }
          frame True {
            # "Result handling for another Command here"
          }
        }
      }
      frame Error {
      }
    }
    n111 = call <extravilib>:"Read.vi"("channel"=w317) -> ("element"=w318:bool)  [unwired: 1 in, 1 out]
  }
  n112 = Unregister For Events(event registration refnum=w13, error in=w12) -> (error out=w7:errorcluster)
  n113 = Merge Errors(w7, w6) -> (w5:errorcluster)
  n114 = Release Notifier(notifier=w4, error in (no error)=w5) -> (error out=w3:errorcluster)  [unwired: 1 in, 2 out]
  n115 = call "Teardown Framework.vi"("error in (no error)"=w3) -> ("error out"=→"error out":errorcluster)  [unwired: 10 in]
